vi "Null Broadcast Events--constant.vi"() -> (3 "FlexiFlowInterface Broadcast Events":T1)   [LabVIEW 2025, in "FlexiFlowInterface.lvlib"]
doc: "Returns the broadcast events cluster with null references for defining the event types in a Register For Events function.\n_____\nCreated using DQMH Event Scripter 7.0.1.1316."
uses:
  FlexiFlowInterface/FlexiFlowInterface.lvlib
  FlexiFlowInterface/Did Init Argument--cluster.ctl
  FlexiFlowInterface/Status Updated Argument--cluster.ctl
  FlexiFlowInterface/Error Reported Argument--cluster.ctl
  FlexiFlowInterface/Stop Argument--cluster.ctl
  FlexiFlowInterface/Get Module Execution Status Argument--cluster.ctl
  FlexiFlowInterface/Device Type--enum.ctl
  <vilib>/Plasmionique/MB Master/MB_Master_TCP/MB_Master_TCP.lvclass
  phlair-shared-libraries/Modbus Flexi-Flow API/Control Mode--enum.ctl
  phlair-shared-libraries/Modbus Flexi-Flow API/Bronkhorst Flexi-Flow ModbusTCP API.lvlib
  phlair-shared-libraries/Modbus Flexi-Flow API/Control Function Values--enum.ctl
  FlexiFlowInterface/Modbus Flexi-Flow Controls--cluster.ctl
  FlexiFlowInterface/Modbus Flexi-Flow Measure State--cluster.ctl
  FlexiFlowInterface/Modbus Flexi-Flow State--cluster.ctl
  FlexiFlowInterface/Broadcast Device States Argument--cluster.ctl
  FlexiFlowInterface/Broadcast State (Data Map) Argument--cluster.ctl
  FlexiFlowInterface/Broadcast Events--cluster.ctl
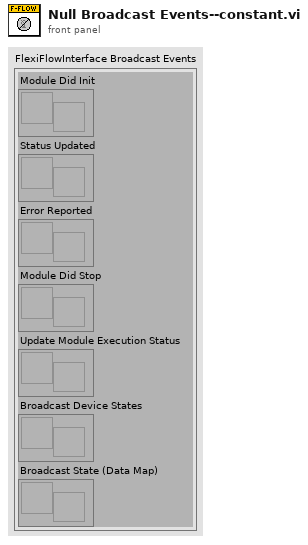
[diagram p1: front panel]
types:
  T1 = typedef "FlexiFlowInterface.lvlib/Broadcast Events--cluster.ctl" = cluster{"Module Did Init":refnum<user-event>, "Status Updated":refnum<user-event>, "Error Reported":refnum<user-event>, "Module Did Stop":refnum<user-event>, "Update Module Execution Status":refnum<user-event>, "Broadcast Device States":refnum<user-event>, "Broadcast State (Data Map)":refnum<user-event>}
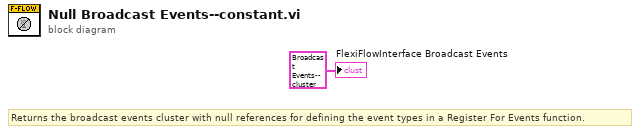
[diagram p0: block diagram]
diagram:
  # "Returns the broadcast events cluster with null references for defining the event types in a Register For Events function."
  "FlexiFlowInterface Broadcast Events" <- T1 {"Module Did Init"=refnum, "Status Updated"=refnum, "Error Reported"=refnum, "Module Did Stop"=refnum, "Update Module Execution Status"=refnum, "Broadcast Device States"=refnum, "Broadcast State (Data Map)"=refnum} ("FlexiFlowInterface Broadcast Events")
